vi "Write-active-item-tag.vi"(8 "error in (no error)":errorcluster, 10 "active.item.tag":string, 11 "dbc in":refnum<class "dbc.lvclass">) -> (0 "error out":errorcluster, 3 "dbc out":refnum<class "dbc.lvclass">)   [LabVIEW 2015, in "dbc.lvclass"]
uses:
  dbc.lvclass
  dbc.lvclass/dbc.ctl
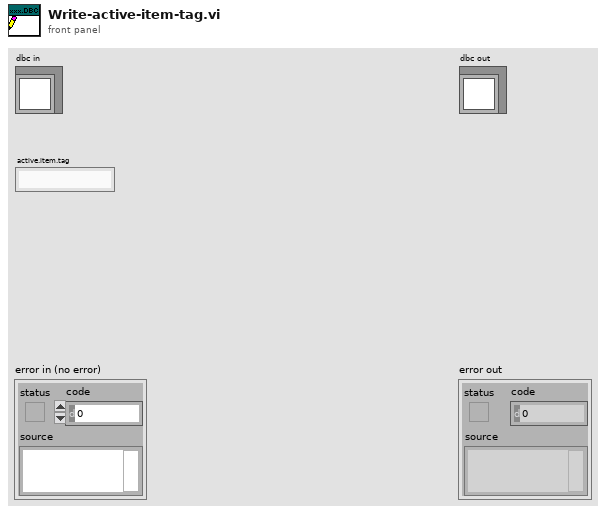
[diagram p1: front panel]
types:
  T1 = typedef "dbc-active-item.ctl" = cluster{"active.frame.tag":string, "activeItemTag":string, "indent.lvl":i32, "symbol":i32}
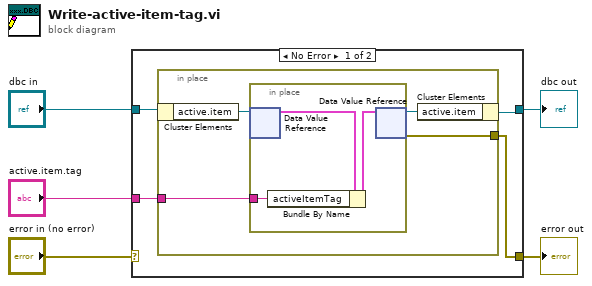
[diagram p0: block diagram]
diagram:
  n1 = case shown="No Error" "error in (no error)" {
    selector: "error in (no error)" -> [_ w17]
    tunnel: [w7 w17] -> w4
    tunnel: [w8 w18] -> w2
    tunnel: "dbc in" -> [w9 w18]
    tunnel: "active.item.tag" -> [w6 _]
    frame No Error {
      n2 = in-place {
        in-place-border: [w11] -> w7
        in-place-border: w6 -> [w10]
        n3 = in-place-cluster #1(w9) -> ("active.item"=w13:refnum<data-value>)
        n4 = in-place {
          in-place-border: w10 -> [w14]
          n5 = in-place-dvr #2(w13) -> (w16:T1)  [unwired: 1 out]
          n6 = Bundle By Name(cluster=w16, "activeItemTag"=w14) -> (w15:T1)
          n7 = in-place-dvr #2(w15) -> (w12:refnum<data-value>, w11:errorcluster)
        }
        n8 = in-place-cluster #1("active.item"=w12) -> (w8:refnum<class "dbc.lvclass">)
      }
    }
    frame Error {
    }
  }
  "error out" <- w4
  "dbc out" <- w2
